vi "Report_Type.vi"(8 "error in (no error)":errorcluster, 11 "IB_CGen in":refnum<class "IB_CGen.lvclass">) -> (0 "error out":errorcluster, 2 "type":string, 3 "IB_CGen out":refnum<class "IB_CGen.lvclass">)   [LabVIEW 2020, in "IB_CGen.lvclass"]
uses:
  <vilib>/AppBuilder/IB_Classes/Source/Container/Build/CGen/IB_CGen.lvclass
  <vilib>/AppBuilder/IB_Classes/Source/Container/Build/CGen/IB_CGen.lvclass/IB_CGen.ctl
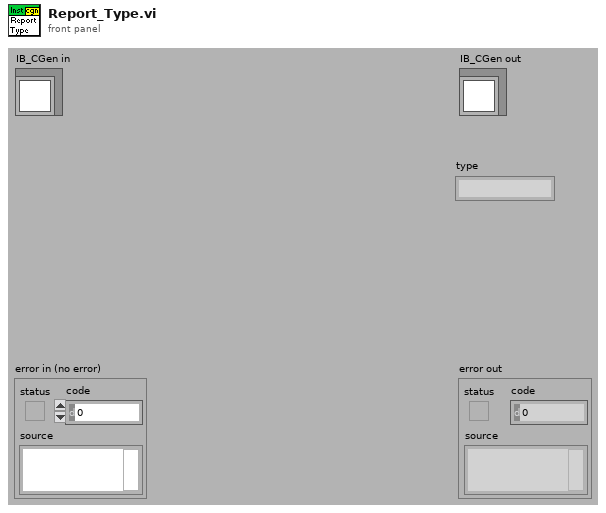
[diagram p1: front panel]
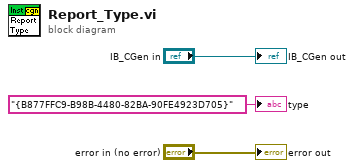
[diagram p0: block diagram]
diagram:
  "error out" <- "error in (no error)"
  "IB_CGen out" <- "IB_CGen in"
  "type" <- "{B877FFC9-B98B-4480-82BA-90FE4923D705}" ("type")
